vi "Drive Get.vi"(7 "Drive Info In":T1, 8 "Show off spin":bool, 9 "Slow Drive":bool, 10 "Y - Axis":dbl, 11 "X - Axis":dbl) -> (3 "Drive Info Out":T1)   [LabVIEW 2013]
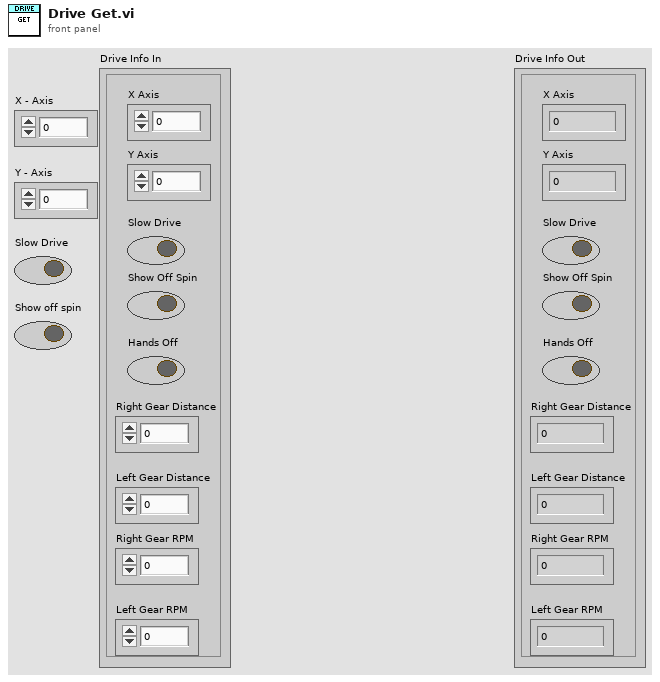
[diagram p1: front panel]
types:
  T1 = cluster{"X Axis":dbl, "Y Axis":dbl, "Slow Drive":bool, "Show Off Spin":bool, "Hands Off":bool, "Right Gear Distance":dbl, "Left Gear Distance ":dbl, "Right Gear RPM":dbl, "Left Gear RPM":dbl}
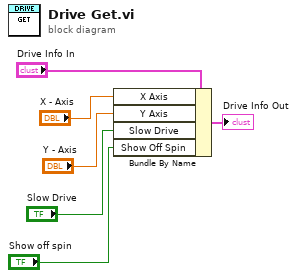
[diagram p0: block diagram]
diagram:
  n1 = Bundle By Name(cluster="Drive Info In", "X Axis"="X - Axis", "Y Axis"="Y - Axis", "Slow Drive"="Slow Drive", "Show Off Spin"="Show off spin") -> (→"Drive Info Out":T1)
